vi "Parse Input.vi"(8 "error in (no error)":errorcluster, 10 "input line":string, 11 "RESP3 Parser in":refnum<class "RESP3 Parser.lvclass">) -> (0 "error out":errorcluster, 1 "RESP3 Value":variant, 2 "finished?":bool, 3 "RESP3 Parser out":refnum<class "RESP3 Parser.lvclass">, 4 "next bytes":i32)   [LabVIEW 2019, in "RESP3.lvlib" / "RESP3 Parser.lvclass"]
doc: "<b>Description</b> Parse a single (\\r\\n delimited) line of RESP3 input and return a valid RESP3 when a value is ready.\n\n<b>Inputs</b>\n<b>input line</b>: A single (\\r\\n terminated) line of input.\n<b>RESP3 Parser in</b>: The previous RESP3 parser state.\n\n<b>Outputs</b>\n<b>RESP3 Parrser out</b>: The updated RESP3 parser state.\n<b>finished?</b>: TRUE if a valid RESP3 is ready.\n<b>RESP3 Value</b>: A valid RESP3 value if 'finished?' is True, otherwise an empty variant.\n\nBSD 3-Clause License\n\nCopyright (c) 2021, TauTerra, LLC\nAll rights reserved.\n\nRedistribution and use in source and binary forms, with or without\nmodification, are permitted provided that the following conditions are met:\n\n1. Redistributions of source code must retain the above copyright notice, this\n list of conditions and the following disclaimer.\n\n2. Redistributions in binary form must reproduce the above copyright notice,\n this list of conditions and the following disclaimer in the documentation\n and/or other materials provided with the distribution.\n\n3. Neither the name of the copyright holder nor the names of its\n contributors may be used to endorse or promote products derived from\n this software without specific prior written permission.\n\nTHIS SOFTWARE IS PROVIDED BY THE COPYRIGHT HOLDERS AND CONTRIBUTORS \"AS IS\"\nAND ANY EXPRESS OR IMPLIED WARRANTIES, INCLUDING, BUT NOT LIMITED TO, THE\nIMPLIED WARRANTIES OF MERCHANTABILITY AND FITNESS FOR A PARTICULAR PURPOSE ARE\nDISCLAIMED. IN NO EVENT SHALL THE COPYRIGHT HOLDER OR CONTRIBUTORS BE LIABLE\nFOR ANY DIRECT, INDIRECT, INCIDENTAL, SPECIAL, EXEMPLARY, OR CONSEQUENTIAL\nDAMAGES (INCLUDING, BUT NOT LIMITED TO, PROCUREMENT OF SUBSTITUTE GOODS OR\nSERVICES; LOSS OF USE, DATA, OR PROFITS; OR BUSINESS INTERRUPTION) HOWEVER\nCAUSED AND ON ANY THEORY OF LIABILITY, WHETHER IN CONTRACT, STRICT LIABILITY,\nOR TORT (INCLUDING NEGLIGENCE OR OTHERWISE) ARISING IN ANY WAY OUT OF THE USE\nOF THIS SOFTWARE, EVEN IF ADVISED OF THE POSSIBILITY OF SUCH DAMAGE."
uses:
  RESP3 Parser.lvclass
  RESP3 Parser.lvclass/RESP3 Parser.ctl
  subVIs/RESP3 Make String Base.vi
  subVIs/get first character.vi
  types/RESP3 data type attribute.vi
  subVIs/RESP3 Make Array Base.vi
  subVIs/strip newline.vi
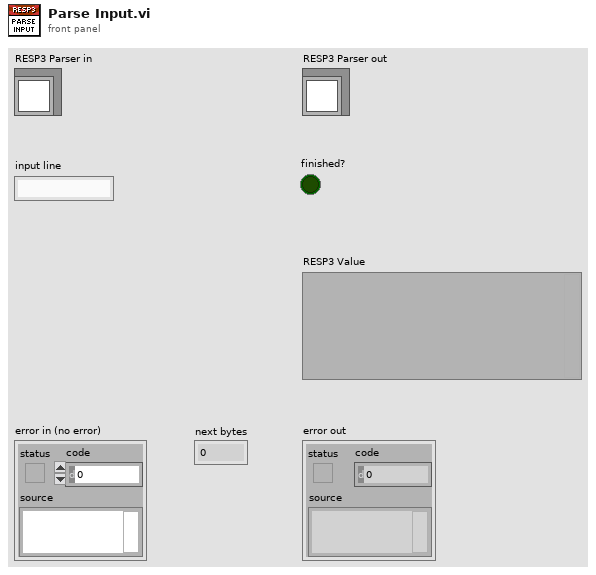
[diagram p1: front panel]
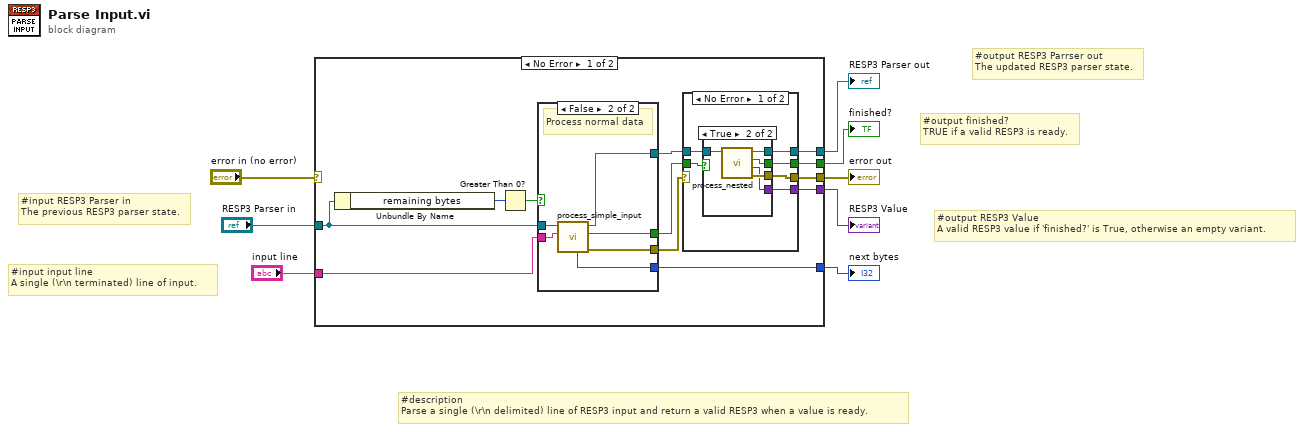
[diagram p0: block diagram]
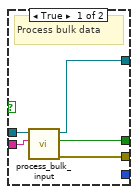
[diagram p4: hidden frame]
diagram:
  # "#output RESP3 Parrser out\nThe updated RESP3 parser state."
  # "#output finished?\nTRUE if a valid RESP3 is ready."
  # "#output RESP3 Value\nA valid RESP3 value if 'finished?' is True, otherwise an empty variant."
  # "#input input line\nA single (\\r\\n terminated) line of input."
  # "#input RESP3 Parser in\nThe previous RESP3 parser state."
  # "#description\nParse a single (\\r\\n delimited) line of RESP3 input and return a valid RESP3 when a value is ready."
  n1 = case shown="No Error" "error in (no error)" {
    selector: "error in (no error)" -> [_ w47]
    tunnel: [w10 w47] -> w7
    tunnel: [w19 w46] -> w6
    tunnel: "RESP3 Parser in" -> [w15 w46]
    tunnel: "input line" -> [w14 _]
    tunnel: [w16 _] -> w3
    tunnel: [w17 _] -> w2
    tunnel: [w9 _] -> w1
    frame No Error {
      n2 = Unbundle By Name(w15) -> ("remaining bytes"=w13:i32)
      n3 = Greater Than 0?(x=w13) -> (x > 0?=w12:bool)
      n4 = case shown="False" w12 {
        tunnel: [w37 w45] -> w20
        tunnel: [w36 w44] -> w18
        tunnel: w15 -> [w38 w43]
        tunnel: w14 -> [w39 w42]
        tunnel: [w35 w41] -> w11
        tunnel: [_ w40] -> w9
        frame True {
          # "Process bulk data"
          n5 = call "process_bulk_input.vi"("input line"=w39, "RESP3 Parser in"=w38) -> ("error out"=w35:errorcluster, "value ready?"=w37:bool, "RESP3 Parser out"=w36:refnum<class "RESP3 Parser.lvclass">)  [unwired: 7 in]
        }
        frame False {
          # "Process normal data"
          n6 = call "process_simple_input.vi"("input line"=w42, "RESP3 Parser in"=w43) -> ("error out"=w41:errorcluster, "value ready?"=w45:bool, "RESP3 Parser out"=w44:refnum<class "RESP3 Parser.lvclass">, "next bytes"=w40:i32)  [unwired: 6 in]
        }
      }
      n7 = case shown="No Error" w11 {
        selector: w11 -> [_ w34]
        tunnel: w20 -> [w26 _]
        tunnel: [w25 w33] -> w19
        tunnel: w18 -> [w24 w33]
        tunnel: [w23 _] -> w17
        tunnel: [w22 _] -> w16
        tunnel: [w21 w34] -> w10
        frame No Error {
          n8 = case shown="True" w26 {
            tunnel: [w27 w31] -> w25
            tunnel: w24 -> [w27 w32]
            tunnel: [_ w30] -> w23
            tunnel: [_ w28] -> w22
            tunnel: [_ w29] -> w21
            frame False {
            }
            frame True {
              n9 = call "process_nested.vi"("RESP3 Parser in"=w32) -> ("error out"=w29:errorcluster, "RESP3 Value"=w28:variant, "value ready?"=w30:bool, "RESP3 Parser out"=w31:refnum<class "RESP3 Parser.lvclass">)  [unwired: 7 in]
            }
          }
        }
        frame Error {
        }
      }
    }
    frame Error {
    }
  }
  "error out" <- w7
  "RESP3 Parser out" <- w6
  "RESP3 Value" <- w3
  "finished?" <- w2
  "next bytes" <- w1
